vi "appendText.vi"(1 "Append?":bool, 2 "Array in":T1(array[cluster])) -> (0 "Array out":T1(array[cluster]))   [LabVIEW 2018]
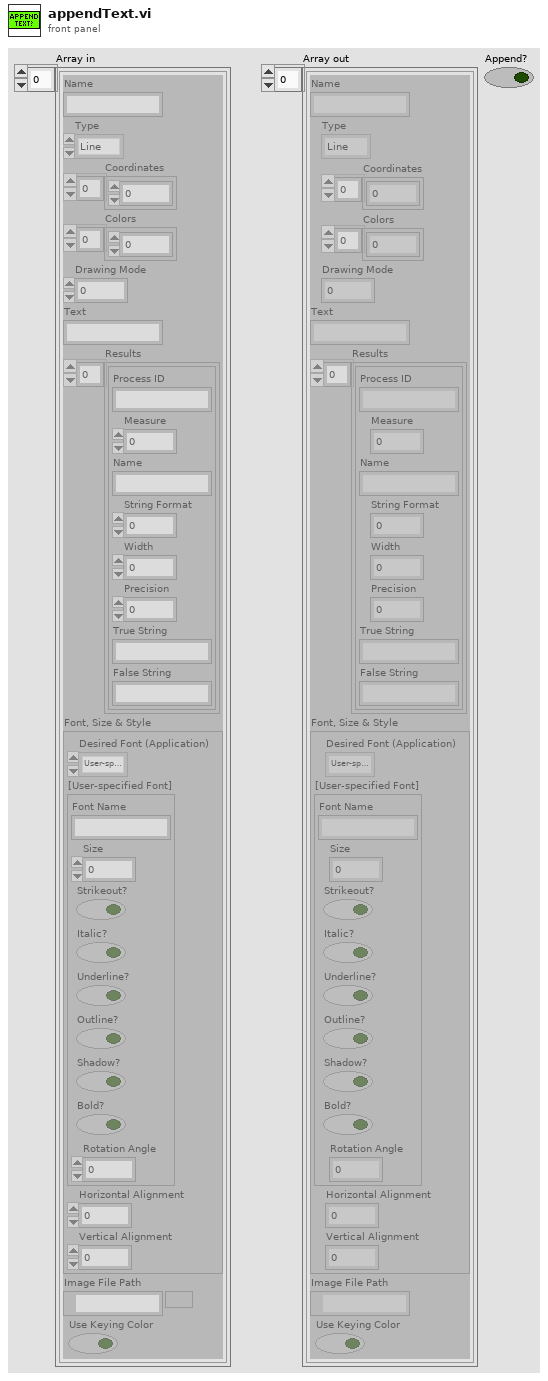
[diagram p1: front panel]
types:
  T1 = cluster{"Name":string, "Type":enum16{"Line", "Broken Line", "Free Hand Line", "Rotated Rectangle", "Oval", "Polygon", "Free Hand", "Bitmap", "Text"}, "Coordinates":i32[], "Colors":u32[], "Drawing Mode":u32, "Text":string, "Results":cluster{"Process ID":string, "Measure":u16, "Name":string, "String Format":u16, "Width":i16, "Precision":i16, "True String":string, "False String":string}[], "Font, Size & Style":cluster{"Desired Font (Application)":enum16{"User-specified Font", "Application Font", "System Font", "Dialog Font"}, "[User-specified Font]":cluster{"Font Name":string, "Size":i16, "Strikeout?":bool, "Italic?":bool, "Underline?":bool, "Outline?":bool, "Shadow?":bool, "Bold?":bool, "Rotation Angle":dbl}, "Horizontal Alignment":i16, "Vertical Alignment":i16}, "Image File Path":path, "Use Keying Color":bool}[]
  T2 = enum16{"Line", "Broken Line", "Free Hand Line", "Rotated Rectangle", "Oval", "Polygon", "Free Hand", "Bitmap", "Text"}
  T3 = cluster{"Name":string, "Type":enum16{"Line", "Broken Line", "Free Hand Line", "Rotated Rectangle", "Oval", "Polygon", "Free Hand", "Bitmap", "Text"}, "Coordinates":i32[], "Colors":u32[], "Drawing Mode":u32, "Text":string, "Results":cluster{"Process ID":string, "Measure":u16, "Name":string, "String Format":u16, "Width":i16, "Precision":i16, "True String":string, "False String":string}[], "Font, Size & Style":cluster{"Desired Font (Application)":enum16{"User-specified Font", "Application Font", "System Font", "Dialog Font"}, "[User-specified Font]":cluster{"Font Name":string, "Size":i16, "Strikeout?":bool, "Italic?":bool, "Underline?":bool, "Outline?":bool, "Shadow?":bool, "Bold?":bool, "Rotation Angle":dbl}, "Horizontal Alignment":i16, "Vertical Alignment":i16}, "Image File Path":path, "Use Keying Color":bool}
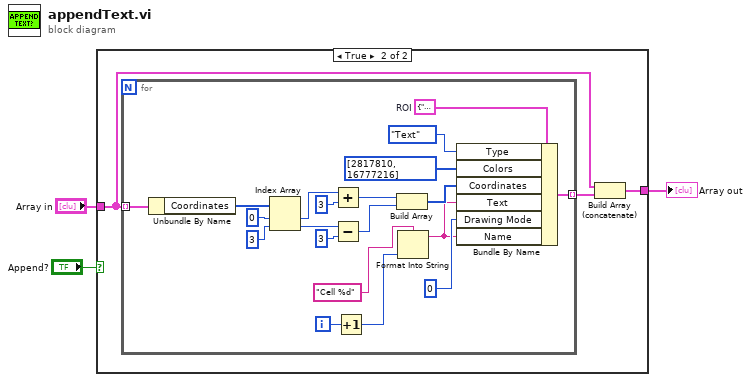
[diagram p0: block diagram]
diagram:
  n1 = case shown="True" "Append?" {
    tunnel: [w4 w7] -> w3
    tunnel: "Array in" -> [w4 w6]
    frame False {
    }
    frame True {
      n2 = for {
        tunnel: w6 -> [w24] mode=indexing
        tunnel: [w8] -> w5 mode=indexing
        i -> [w11]
        w27 = T3 {"Name"="", "Type"=enum."Text", "Coordinates"=[], "Colors"=[2817810], "Drawing Mode"=0, "Text"="", "Results"=[], "Font, Size & Style"={"Desired Font (Application)"=enum."System Font", "[User-specified Font]"={"Font Name"="Tahoma", "Size"=13, "Strikeout?"=FALSE, "Italic?"=FALSE, "Underline?"=FALSE, "Outline?"=FALSE, "Shadow?"=FALSE, "Bold?"=FALSE, "Rotation Angle"=0.0}, "Horizontal Alignment"=0, "Vertical Alignment"=0}, "Image File Path"=path "", "Use Keying Color"=FALSE}  # ROI
        n3 = Unbundle By Name(w24) -> ("Coordinates"=w23:i32[])
        n4 = Index Array(array=w23, index #1=0 ("index"), index #2=3 ("index")) -> (element #1=w20:i32, element #2=w18:i32)
        n5 = Add(x=w20, y=3) -> (x+y=w16:i32)
        n6 = Subtract(x=w18, y=3) -> (x-y=w15:i32)
        n7 = Increment(x=w11) -> (x+1=w12:i32)
        n8 = Build Array(w16, w15) -> (w14:i32[])
        n9 = Format Into String(format string="Cell %d", w12) -> (resulting string=w9:string)  [unwired: 2 in, 1 out]
        n10 = Bundle By Name(cluster=w27, "Type"=T2."Text", "Colors"=u32[] [2817810, 16777216], "Coordinates"=w14, "Text"=w9, "Drawing Mode"=u32 0, "Name"=w9) -> (w8:T3)
      }
      n11 = Build Array (concatenate)(w6, w5) -> (w7:T1)
    }
  }
  "Array out" <- w3
